vi "ATF-Pump-AI_V_Read.vi"(7 "Data FIFO Ref":T1, 8 "error in":errorcluster, 10 "number of samples per channel":i32=51, 11 "AI_V_Task":refnum<k21>) -> (0 "error out":errorcluster, 3 "AI_V_Task":refnum<k21>)   [LabVIEW 2022 SP3]
uses:
  RT Controls/ATF-Pump-Data FIFO.ctl
  <vilib>/DAQmx/read.llb/DAQmx Read (Analog 1D Wfm NChan NSamp).vi
  <vilib>/DAQmx/miscellaneous.llb/DAQmx Fill In Error Info.vi
  <vilib>/measure/madcrms.llb/Averaged DC-RMS for N Chan.vi
  <vilib>/measure/NI_MAPro.lvlib
panel:
  out "y":u32
  out "overflow? 2":bool
  out "overflow?":bool
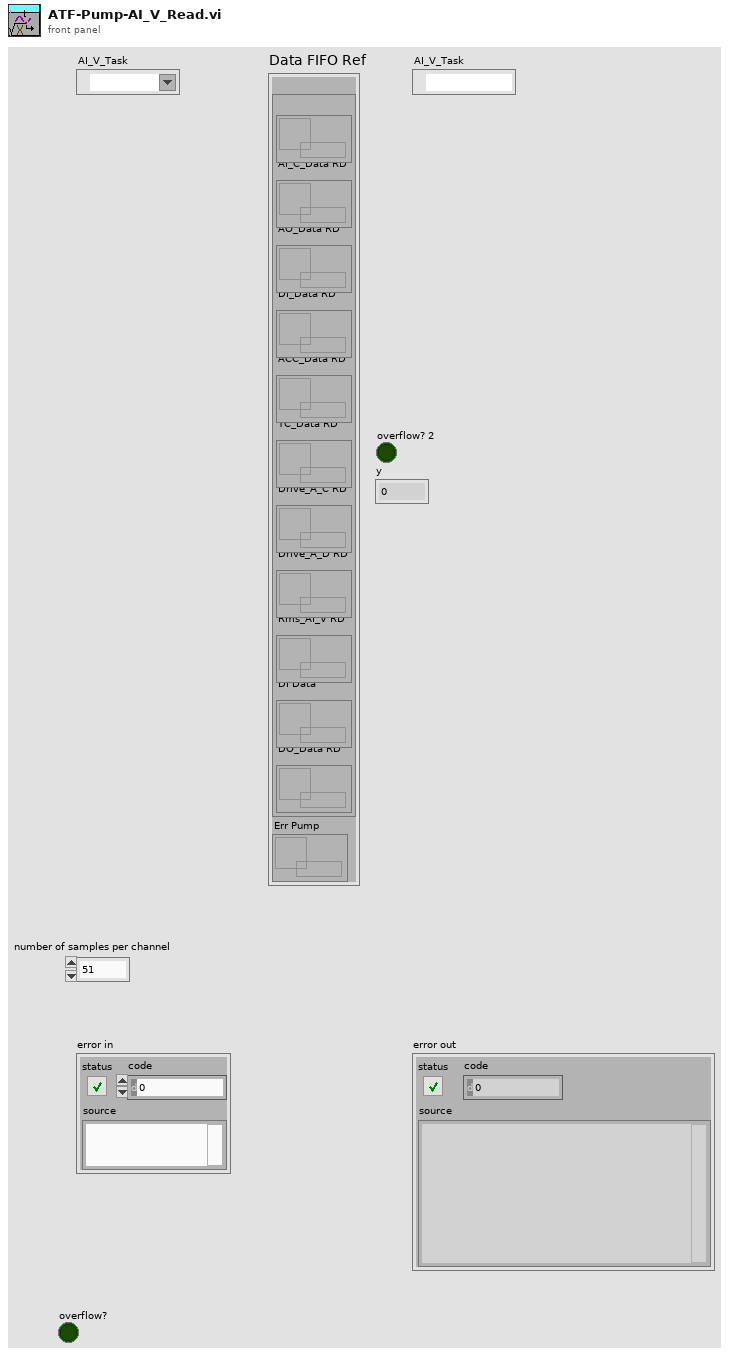
[diagram p1: front panel]
types:
  T1 = typedef "ATF-Pump-Data FIFO.ctl" = cluster{"RD":cluster{"AI_V_Data RD":refnum<queue>, "AI_C_Data RD":refnum<queue>, "AO_Data RD":refnum<queue>, "DI_Data RD":refnum<queue>, "ACC_Data RD":refnum<queue>, "TC_Data RD":refnum<queue>, "Drive_A_C RD":refnum<queue>, "Drive_A_D RD":refnum<queue>, "Rms_AI_V RD":refnum<queue>, "DI Data":refnum<queue>, "DO_Data RD":refnum<queue>}, "Err Pump":refnum<queue>}
  T2 = enum16{"AI C", "AI V", "AO", "DI", "DO", "TC", "ACC", "RT PMP", "DR A"}
  T3 = cluster{"window for DC":enum16{"Rectangular (none)", "Hanning", "Low side lobe"}, "output function":enum16{"DC only", "RMS only", "DC and RMS"}, "window for RMS":enum16{"Rectangular (none)", "Hanning", "Low side lobe"}, "exp. time constant":dbl, "Ignore input start time":bool}
  T4 = enum16{"Init", "Read 'All'", "Read 'n'", "Read '1'", "Write '1'", "Write 'n'", "Write 'All'"}
  T5 = cluster{"Start DAQ":bool, "Stop DAQ":bool, "RT Stop":bool, "RT Exit":bool, "Start Seq":bool}
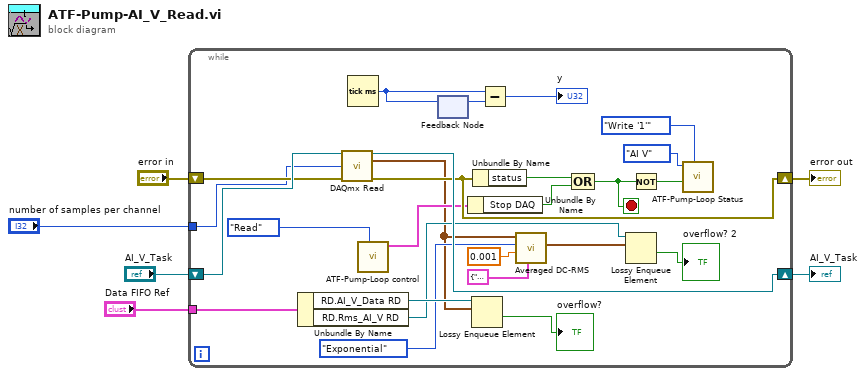
[diagram p0: block diagram]
diagram:
  n1 = while {
    shift-right: [w30] -> w1
    shift-left: "AI_V_Task" -> [w32]
    shift-right: [w29] -> w4
    shift-left: "error in" -> [w31]
    tunnel: "number of samples per channel" -> [w14]
    tunnel: "Data FIFO Ref" -> [w23]
    stop <- w28 stop-if-true
    n2 = Unbundle By Name(w23) -> ("RD.AI_V_Data RD"=w20:refnum<queue>, "RD.Rms_AI_V RD"=w13:refnum<queue>)
    n3 = call-poly <vilib>:"DAQmx Read.vi"("task/channels in"=w32, "number of samples per channel"=w14, "error in"=w31) -> ("task out"=w30:refnum<k21>, "data"=w11:waveform(dbl)[], "error out"=w29:errorcluster)  [unwired: 10 in]
    n4 = Tick Count (ms)() -> (millisecond timer value=w9:u32)
    n5 = call "ATF-Pump-Loop control.vi"("Action"=enum16{"Init", "Write", "Read"}."Read") -> ("Loop Control out"=w26:T5)  [unwired: 9 in, 1 out]
    n6 = feedback-in #1(w9) -> ()
    n7 = feedback #1() -> (w8:u32)  [unwired: 1 in]
    n8 = Unbundle By Name(w26) -> ("Stop DAQ"=w25:bool)
    n9 = Lossy Enqueue Element(queue=w20, element=w11) -> (overflow?=→"overflow?":bool)  [unwired: 1 in, 3 out]
    n10 = Unbundle By Name(w29) -> ("status"=w27:bool)
    n11 = Subtract(x=w9, y=w8) -> (x-y=→"y":u32)
    n12 = call-poly <vilib>:"Averaged DC-RMS.vi"("averaging control"=T3 {"window for DC"=enum."Rectangular (none)", "output function"=enum."RMS only", "window for RMS"=enum."Rectangular (none)", "exp. time constant"=-1.0, "Ignore input start time"=FALSE}, "averaging time"=0.001, "averaging type"=enum16{"Linear", "Exponential"}."Exponential", "signals in"=w11) -> ("RMS value waveforms"=w12:waveform(dbl)[])  [unwired: 3 in, 4 out]
    n13 = Compound Arithmetic op=OR(w27, w25) -> (w28:bool)
    n14 = Lossy Enqueue Element(queue=w13, element=w12) -> (overflow?=→"overflow? 2":bool)  [unwired: 1 in, 3 out]
    n15 = Not(x=w28) -> (.not. x?=w21:bool)
    n16 = call "ATF-Pump-Loop Status.vi"("Option"=T4."Write '1'", "Status"=w21, "Loop"=T2."AI V") -> ()  [unwired: 6 in, 3 out]
  }
  "error out" <- w4
  "AI_V_Task" <- w1
